vi "Timebase_DELay.vi"(7 "Write?":bool, 8 "Error":errorcluster caption="错误输入（无错误）", 10 "Time(s)":dbl, 11 "VISA resource name":refnum<visa-resource-name>) -> (0 "Error out":errorcluster, 2 "Time out(s)":dbl, 3 "VISA resource name out":refnum<visa-resource-name>)   [LabVIEW 2020]
doc: "延时时间"
panel:
  out "读取缓冲区":string
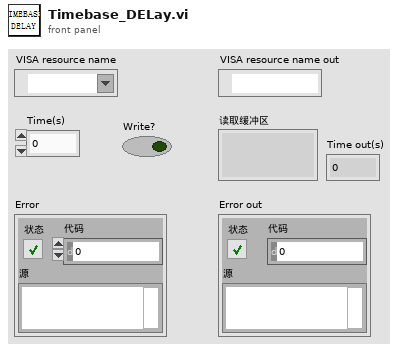
[diagram p1: front panel]
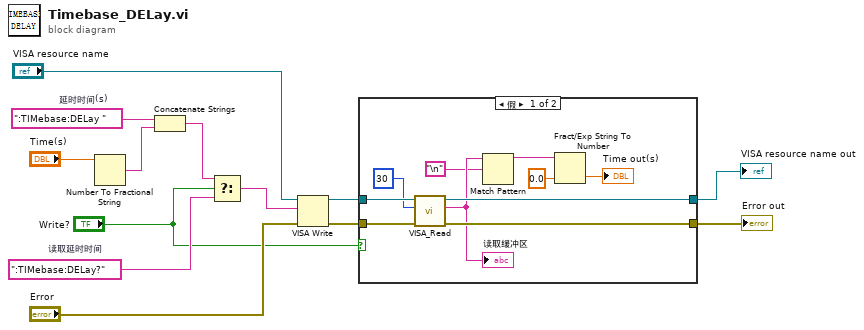
[diagram p0: block diagram]
diagram:
  w8 = ":TIMebase:DELay?"  # 读取延时时间
  w12 = ":TIMebase:DELay "  # 延时时间(s)
  n1 = Number To Fractional String(number="Time(s)") -> (F-format string=w11:string)  [unwired: 3 in]
  n2 = Concatenate Strings(w12, w11) -> (w9:string)
  n3 = Select(t=w9, s="Write?", f=w8) -> (s? t:f=w7:string)
  n4 = VISA Write(VISA resource name="VISA resource name", write buffer=w7, error in (no error)="Error") -> (VISA resource name out=w3:refnum<visa-resource-name>, error out=w5:errorcluster)  [unwired: 1 out]
  n5 = case shown="假" "Write?" {
    tunnel: w3 -> [w23 w25]
    tunnel: w5 -> [w22 w24]
    tunnel: [w20 w24] -> w4
    tunnel: [w21 w25] -> w1
    frame False {
      n6 = call "VISA_Read.vi"("Error"=w22, "字节总数"=u32 30, "VISA resource name"=w23) -> ("Error out"=w20:errorcluster, "读取缓冲区"=w19:string, "VISA resource name out"=w21:refnum<visa-resource-name>)  [unwired: 6 in]
      "读取缓冲区" <- w19
      n7 = Match Pattern(string=w19, regular expression="\n") -> (before substring=w16:string)  [unwired: 1 in, 3 out]
      n8 = Fract/Exp String To Number(string=w16, default (0 dbl)=0.0 ("默认(0 I32)")) -> (number=→"Time out(s)":dbl)  [unwired: 2 in, 1 out]
    }
    frame True {
    }
  }
  "VISA resource name out" <- w1
  "Error out" <- w4
